vi "Get.vi"(8 "error in":errorcluster, 10 "endPoint":string, 11 "firebase in":refnum<class "firebase.lvclass">) -> (0 "error out":errorcluster, 2 "Json String":string, 3 "firebase out":refnum<class "firebase.lvclass">)   [LabVIEW 2019, in "firebase.lvclass"]
uses:
  firebase.lvclass
  <vilib>/NI/Advanced HTTP Client/Session.lvclass
  <vilib>/NI/Advanced HTTP Client/Header--Combo Box.ctl
  Error Message--cluster.ctl
  8b64f89a-9e96-43c3-a012-814e780b19c4.vi
  <vilib>/JDP Science/JSONtext/JSONtext.lvlib
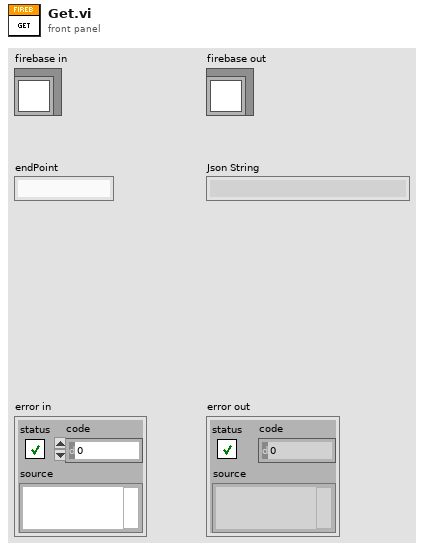
[diagram p1: front panel]
types:
  T1 = typedef "lib_NI_Advanced HTTP Client.lvlib/Session.lvclass/Header--Combo Box.ctl" = string
  T2 = typedef "firebase.lvclass/Success Sign In--cluster.ctl" = cluster{"kind":string, "idToken":string, "email":string, "refreshToken":string, "expiresIn":string, "localId":string, "displayName":string, "registered":bool}
  T3 = typedef "firebase.lvclass/Error Message--cluster.ctl" = cluster{"error":cluster{"code":i32, "message":string, "errors":cluster{"message":string, "domain":string, "reason":string}[]}}
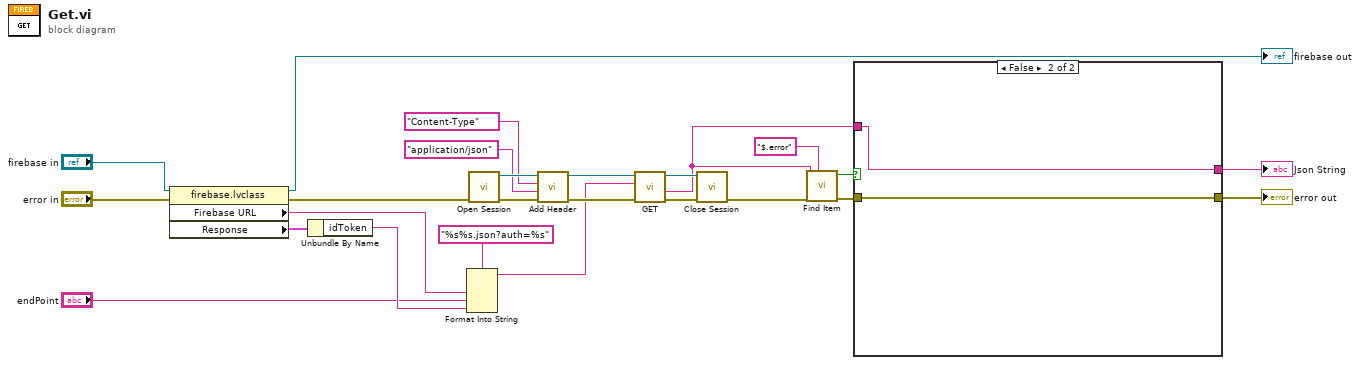
[diagram p0: block diagram]
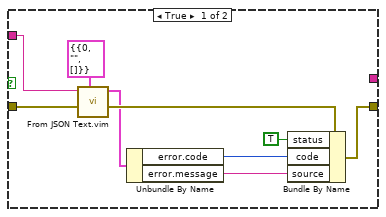
[diagram p2: hidden frame]
diagram:
  n1 = property class="firebase.lvclass"(reference="firebase in", error in="error in") -> (reference out=→"firebase out":refnum<class "firebase.lvclass">, error out=w20:errorcluster, "Firebase URL"=w15:string, "Response"=w4:T2)
  n2 = Unbundle By Name(w4) -> ("idToken"=w3:string)
  n3 = Format Into String(format string="%s%s.json?auth=%s", w15, "endPoint", w3) -> (resulting string=w8:string)  [unwired: 2 in, 1 out]
  n4 = call <vilib>:"Open Session.vi"("error in"=w20) -> ("error out"=w23:errorcluster, "session"=w12:refnum<class "Session.lvclass">)  [unwired: 9 in]
  n5 = call <vilib>:"Add Header.vi"("error in"=w23, "value"="application/json", "header"=T1 "Content-Type", "session in"=w12) -> ("error out"=w22:errorcluster, "session out"=w11:refnum<class "Session.lvclass">)  [unwired: 6 in]
  n6 = call <vilib>:"GET.vi"("error in"=w22, "url"=w8, "session in"=w11) -> ("error out"=w24:errorcluster, "body"=w5:string, "session out"=w13:refnum<class "Session.lvclass">)  [unwired: 4 in, 2 out]
  n7 = call <vilib>:"Close Session.vi"("error in"=w24, "session"=w13) -> ("error out"=w19:errorcluster)  [unwired: 9 in]
  n8 = call <vilib>:"Find Item.vi"("$Path or Item Name"="$.error", "error in (no error)"=w19, "JSON"=w5) -> ("error out"=w21:errorcluster, "Found"=w6:bool)  [unwired: 5 in, 2 out]
  n9 = case shown="False" w6 {
    tunnel: [w32 w36] -> w18
    tunnel: w21 -> [w34 w36]
    tunnel: w5 -> [w30 w35]
    tunnel: [_ w35] -> w1
    frame True {
      n10 = call "From JSON Text.vim"("Data Type and Default Value"=T3 {"error"={"code"=0, "message"="", "errors"=[]}} ("Error Message"), "error in (no error)"=w34, "JSON"=w30) -> ("error out"=w33:errorcluster, "Data out"=w29:T3)  [unwired: 7 in]
      n11 = Unbundle By Name(w29) -> ("error.code"=w28:i32, "error.message"=w27:string)
      n12 = Bundle By Name(cluster=w33, "status"=TRUE, "code"=w28, "source"=w27) -> (w32:errorcluster)
    }
    frame False {
    }
  }
  "error out" <- w18
  "Json String" <- w1
